vi "DB_ActualizaEstadoEquipos.vi"(10 "ESTADO_EQUIPO":string, 11 "NOMBRE_EQUIPO":string) -> (0 "error out":errorcluster)   [LabVIEW 2018]
uses:
  <vilib>/addons/database/Connection.llb/DB Tools Open Connec (Path).vi
  <vilib>/addons/database/Connection.llb/Conn Execute.vi
  <vilib>/addons/database/Recordset.llb/Rec Fetch Recordset Data (R).vi
  <vilib>/addons/database/Recordset.llb/Rec Destroy - Connection.vi
  <vilib>/addons/database/NI_Database_API.lvlib
panel:
  in  "error in (no error)":errorcluster
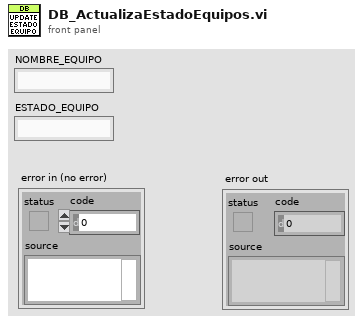
[diagram p1: front panel]
types:
  T1 = typedef "NI_Database_API.lvlib/Conn ObjectReference.ctl" = refnum<k1>
  T2 = typedef "NI_Database_API.lvlib/Rec ObjectReference.ctl" = refnum<k1>
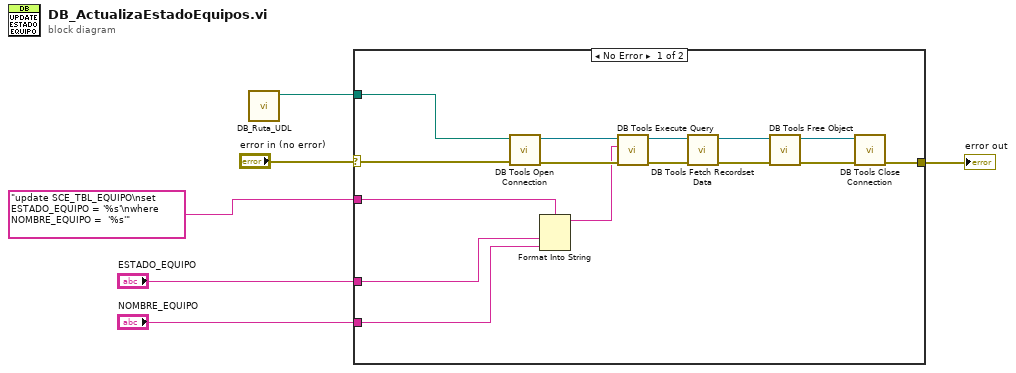
[diagram p0: block diagram]
diagram:
  n1 = call "DB_Ruta_UDL.vi"() -> ("UDL ruta"=w1:path)  [unwired: 11 in]
  n2 = case shown="No Error" "error in (no error)" {
    selector: "error in (no error)" -> [w16 w22]
    tunnel: [w18 w22] -> w6
    tunnel: "update SCE_TBL_EQUIPO\nset ESTADO_EQUIPO = '%s'\nwhere NOMBRE_EQUIPO =  '%s'" ("SQL") -> [w12 _]
    tunnel: "ESTADO_EQUIPO" -> [w11 _]
    tunnel: "NOMBRE_EQUIPO" -> [w10 _]
    tunnel: w1 -> [w8 _]
    frame No Error {
      n3 = call-poly <vilib>:"DB Tools Open Connection.vi"("error in (no error)"=w16, "connection information"=w8) -> ("error out"=w21:errorcluster, "connection reference"=w19:T1)  [unwired: 6 in]
      n4 = Format Into String(format string=w12, w11, w10) -> (resulting string=w9:string)  [unwired: 2 in, 1 out]
      n5 = call-poly <vilib>:"DB Tools Execute Query.vi"("error in (no error)"=w21, "SQL query"=w9, "connection reference"=w19) -> ("error out"=w17:errorcluster, "recordset reference"=w15:T2)  [unwired: 5 in]
      n6 = call-poly <vilib>:"DB Tools Fetch Recordset Data.vi"("error in (no error)"=w17, "recordset reference"=w15) -> ("error out"=w13:errorcluster, "recordset reference out"=w14:T2)  [unwired: 3 in, 1 out]
      n7 = call-poly <vilib>:"DB Tools Free Object.vi"("error in (no error)"=w13, "recordset reference"=w14) -> ("error out"=w20:errorcluster, "connection reference"=w7:T1)  [unwired: 8 in]
      n8 = call <vilib>:"DB Tools Close Connection.vi"("error in (no error)"=w20, "connection reference"=w7) -> ("error out"=w18:errorcluster)  [unwired: 5 in]
    }
    frame Error {
    }
  }
  "error out" <- w6
